vi "Read Array of Move Button Configurations.vi"(11 "VacuumLine in":refnum<class "VacuumLine.lvclass">) -> (2 "Array of Move Button Configurations":T1[](array[typedef]) {"Target pos" format="%#_f mm"}, 3 "VacuumLine out":refnum<class "VacuumLine.lvclass">)   [LabVIEW 2016, in "Hardware.lvlib" / "VacuumLine.lvlib" / "VacuumLine.lvclass"]
uses:
  <userlib>/Common Components/Hardware/Abstract System/VacuumLine/VacuumLine/VacuumLine.lvclass
  <userlib>/Common Components/Hardware/Abstract System/VacuumLine/VacuumLine/Button Config Cluster.ctl
  <userlib>/Common Components/Hardware/Abstract System/VacuumLine/VacuumLine/VacuumLine.lvclass/VacuumLine.ctl
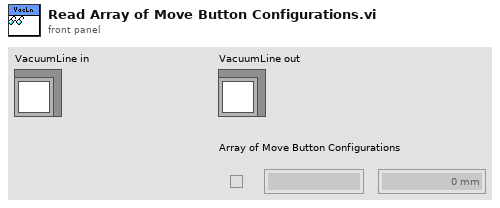
[diagram p1: front panel]
types:
  T1 = typedef "Hardware.lvlib/VacuumLine.lvlib/VacuumLine.lvclass/Button Config Cluster.ctl" = cluster{"Enabled?":bool, "Text on button":string, "Target pos":dbl}
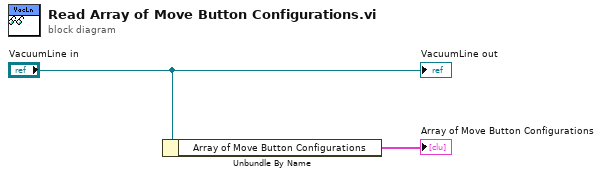
[diagram p0: block diagram]
diagram:
  n1 = Unbundle By Name("VacuumLine in") -> ("Array of Move Button Configurations"=→"Array of Move Button Configurations":T1[])
  "VacuumLine out" <- "VacuumLine in"
